vi "LesserTest.vi"() -> ()   [LabVIEW 2016, in "test_AssertControlValue.lvlib"]
uses:
  test_AssertControlValue.lvlib
  main/apis/Setup/GetVI/GetVIByPath.vi
  main/apis/Stimulus/ValueSignal/ValueSignalByPathString.vi
  main/apis/Assert/AssertControlValue/Less.vi
  main/apis/Setup/GetVI/GetVI.lvlib
  <vilib>/addons/_JKI Toolkits/Caraya/classes/Test/Test.lvclass
  main/apis/Assert/AssertControlValue/AssertControlValue.lvlib
panel:
  out "error out":errorcluster
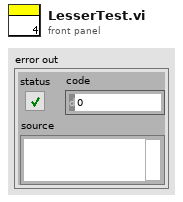
[diagram p1: front panel]
types:
  T1 = enum32{"Invalid", "Standard", "Closed", "Hidden", "Minimized", "Maximized"}
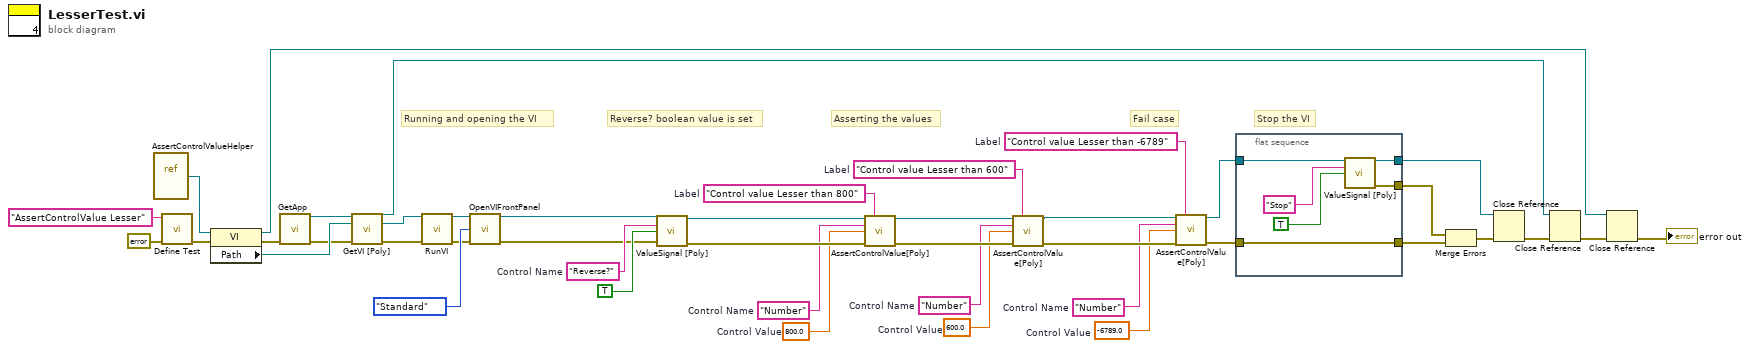
[diagram p0: block diagram]
diagram:
  w2 = "Control value Lesser than -6789"  # Label
  w3 = "Control value Lesser than 600"  # Label
  w4 = "Control value Lesser than 800"  # Label
  w20 = -6789.0  # Control Value
  w21 = "Number"  # Control Name
  w24 = 600.0  # Control Value
  w25 = "Number"  # Control Name
  w28 = 800.0  # Control Value
  w29 = "Number"  # Control Name
  w39 = "Reverse?"  # Control Name
  # "Reverse? boolean value is set"
  # "Running and opening the VI"
  # "Asserting the values"
  # "Stop the VI"
  # "Fail case"
  n1 = vi-ref "AssertControlValueHelper.vi"() -> (w33:refnum<vi>)
  n2 = call <vilib>:"Define Test.vi"("error in (no error)"=errorcluster {"status"=FALSE, "code"=0, "source"=""}, "Label (VI Title)"="AssertControlValue Lesser") -> ("error out"=w34:errorcluster)  [unwired: 9 in]
  n3 = property on="Property Node" class="VI"(reference=w33, error in=w34) -> (reference out=w5:refnum<vi>, error out=w42:errorcluster, "Path"=w41:path)
  n4 = call "GetApp.vi"("error in (no error)"=w42) -> ("Application Ref"=w43:refnum<vi>, "error out"=w40:errorcluster)  [unwired: 13 in]
  n5 = call-poly "GetVI [Poly].vi"("Application Ref in"=w43, "VI Path"=w41, "error in (no error)"=w40) -> ("Application Ref out"=w6:refnum<vi>, "VI Reference"=w37:refnum<vi>, "error out"=w36:errorcluster)  [unwired: 10 in]
  n6 = call "RunVI.vi"("VI Reference In"=w37, "error in"=w36) -> ("VI Reference Out"=w8:refnum<vi>, "error out"=w9:errorcluster)  [unwired: 12 in]
  n7 = call "OpenVIFrontPanel.vi"("VI Reference In"=w8, "State(Standard)"=T1."Standard", "error in"=w9) -> ("VI Reference Out"=w12:refnum<vi>, "error out"=w11:errorcluster)  [unwired: 11 in]
  n8 = call-poly "ValueSignal [Poly].vi"("VI Reference In"=w12, "Control Name"=w39, "Value (Signaling)"=TRUE, "error in"=w11) -> ("VI Reference Out"=w30:refnum<vi>, "error out"=w31:errorcluster)  [unwired: 10 in]
  n9 = call-poly "AssertControlValue[Poly].vi"("VI Reference In"=w30, "Label"=w4, "Control Name"=w29, "Control Value"=w28, "Error In"=w31) -> ("VI Reference Out"=w27:refnum<vi>, "Error Out"=w26:errorcluster)  [unwired: 9 in]
  n10 = call-poly "AssertControlValue[Poly].vi"("VI Reference In"=w27, "Label"=w3, "Control Name"=w25, "Control Value"=w24, "Error In"=w26) -> ("VI Reference Out"=w22:refnum<vi>, "Error Out"=w23:errorcluster)  [unwired: 9 in]
  n11 = call-poly "AssertControlValue[Poly].vi"("VI Reference In"=w22, "Label"=w2, "Control Name"=w21, "Control Value"=w20, "Error In"=w23) -> ("VI Reference Out"=w19:refnum<vi>, "Error Out"=w17:errorcluster)  [unwired: 9 in]
  n12 = flat-sequence {
    tunnel: w19 -> [w47]
    tunnel: [w46] -> w18
    tunnel: w17 -> [w45]
    tunnel: [w45] -> w16
    tunnel: [w44] -> w13
    frame #0 {
      n13 = call-poly "ValueSignal [Poly].vi"("VI Reference In"=w47, "Control Name"="Stop" ("Class Name"), "Value (Signaling)"=TRUE) -> ("VI Reference Out"=w44:refnum<vi>, "error out"=w46:errorcluster)  [unwired: 11 in]
    }
  }
  n14 = Merge Errors(w18, w16) -> (w15:errorcluster)
  n15 = Close Reference(reference=w13, error in (no error)=w15) -> (error out=w14:errorcluster)
  n16 = Close Reference(reference=w6, error in (no error)=w14) -> (error out=w7:errorcluster)
  n17 = Close Reference(reference=w5, error in (no error)=w7) -> (error out=→"error out":errorcluster)
